vi "Write String.vi"(7 "count (-1: all)":i64=-1 format="%d elements", 8 "error in (no error)":errorcluster, 9 "offset (0)":u64 format="%d bytes", 10 "buffer in":string, 11 "Pointer in":refnum<class "Pointer.lvclass">) -> (0 "error out":errorcluster, 1 "offset + size":u64 format="%d bytes", 2 "buffer out":string, 3 "Pointer out":refnum<class "Pointer.lvclass">)   [LabVIEW 2017, in "Memory Manager.lvlib" / "Pointer.lvclass"]
doc: "Writes <b>count</b> elements from the provided <b>buffer</b> to the address specified by <b>pointer + offset</b>."
uses:
  Pointer.lvclass
  Write (No Check) String.vi
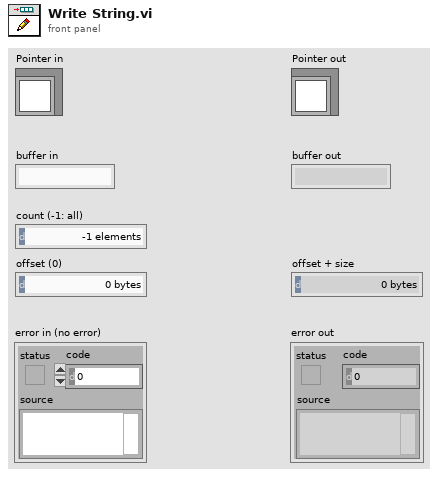
[diagram p1: front panel]
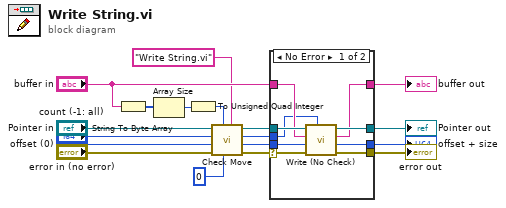
[diagram p0: block diagram]
diagram:
  n1 = String To Byte Array(string="buffer in") -> (unsigned byte array=w18:u8[])
  n2 = Array Size(array=w18) -> (size(s)=w17:i32)
  n3 = To Unsigned Quad Integer(1:w17) -> (0:w12:u64)
  n4 = call "Check Move.vi"("source vi name"="Write String.vi", "count power of 2"=i16 0, "buffer count"=w12, "error in (no error)"="error in (no error)", "offset (0)"="offset (0)", "move count (-1: rest)"="count (-1: all)", "Pointer in"="Pointer in") -> ("error out"=w15:errorcluster, "offset"=w14:u64, "count"=w13:u64, "Pointer out"=w16:refnum<class "Pointer.lvclass">)  [unwired: 1 in]
  n5 = case shown="No Error" w15 {
    selector: w15 -> [w27 w30]
    tunnel: w16 -> [w25 w29]
    tunnel: w14 -> [w26 w31]
    tunnel: "buffer in" -> [w20 w28]
    tunnel: [w24 w30] -> w7
    tunnel: [w23 w29] -> w8
    tunnel: [w22 w31] -> w2
    tunnel: [w21 w28] -> w5
    tunnel: w13 -> [w19 _]
    frame No Error {
      n6 = call-poly "Write (No Check).vi"("count"=w19, "error in (no error)"=w27, "offset (0)"=w26, "buffer in"=w20, "Pointer in"=w25) -> ("error out"=w24:errorcluster, "offset + size"=w22:u64, "buffer out"=w21:string, "Pointer out"=w23:refnum<class "Pointer.lvclass">)  [unwired: 3 in]
    }
    frame Error {
    }
  }
  "error out" <- w7
  "Pointer out" <- w8
  "buffer out" <- w5
  "offset + size" <- w2
